vi "arm control.vi"(1 "State":T1, 2 "Z Axis (Tuning)":dbl) -> (0 "setpoint":dbl format="%.2f")   [LabVIEW 2013]
uses:
  typedefs/fg_typedef.ctl
  typedefs/subStates.ctl
panel:
  in  "lower limit":dbl=-0.015 format="%#_13g"
  in  "upper limit":dbl=0.015 format="%#_13g"
  in  "Up Setpoint":dbl format="%#_13g"
  # "Things needing Tuning"
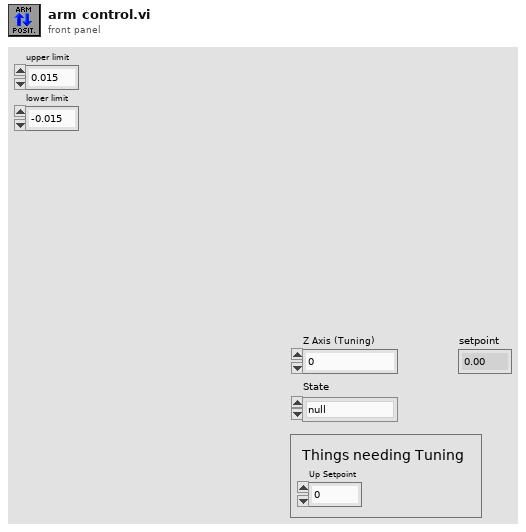
[diagram p1: front panel]
types:
  T1 = typedef "subStates.ctl" = enum16{"null", "wait", "driver control", "auto", "manual override", "hold position", "rotate", "pickup", "pass", "load", "goto shoot", "shoot high goal", "shoot low goal", "cancel arm", "cancel shooter", "end"}
  T2 = typedef "fg_typedef.ctl" = enum16{"Get", "Set"}
  T3 = typedef "WPI_DigitalInputDevRef.ctl" = cluster{"DevStatus":errorcluster, "DIO Channel":T4, "Digital Module":T5}
  T4 = typedef "FPGA_DIOChannel.ctl" = enum8{"DIO 1", "DIO 2", "DIO 3", "DIO 4", "DIO 5", "DIO 6", "DIO 7", "DIO 8", "DIO 9", "DIO 10", "DIO 11", "DIO 12", "DIO 13", "DIO 14", "Invalid"}
  T5 = typedef "FPGA_TypedefDigitalModule.ctl" = enum16{"Digital Module 1", "Digital Module 2"}
  T6 = typedef "WPI_EncoderDevRef.ctl" = cluster{"DevStatus":errorcluster, "EncoderIndex":T7, "CounterIndex":T8, "DistancePerCount":dbl, "Decoding Type":T9}
  T7 = typedef "FPGA_EncoderIdx.ctl" = enum8{"Enc 0", "Enc 1", "Enc 2", "Enc 3", "Invalid"}
  T8 = typedef "FPGA_CounterCtrSystemIndex.ctl" = enum8{"Ctr 0", "Ctr 1", "Ctr 2", "Ctr 3", "Ctr 4", "Ctr 5", "Ctr 6", "Ctr 7", "Invalid"}
  T9 = typedef "WPI_EncoderType.ctl" = enum16{"1x", "2x", "4x"}
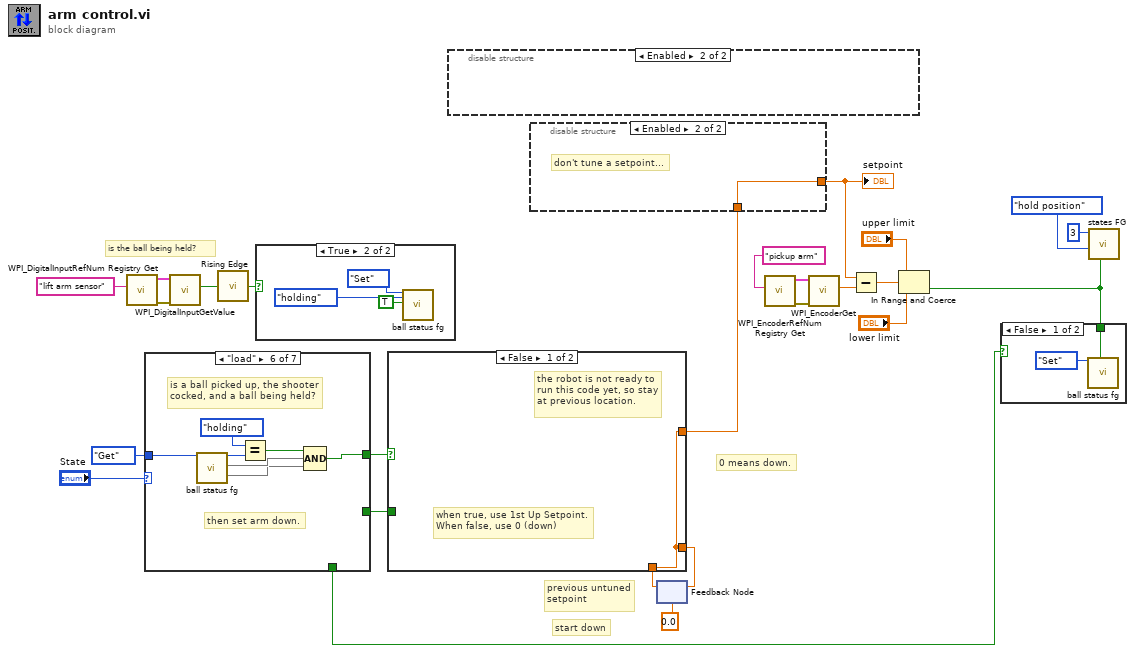
[diagram p0: block diagram]
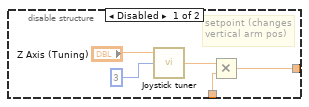
[diagram p3: hidden frame]
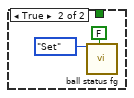
[diagram p4: hidden frame]
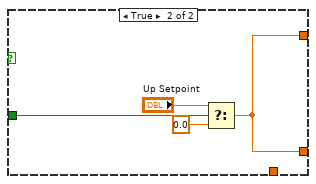
[diagram p6: hidden frame]
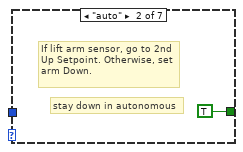
[diagram p8: hidden frame]
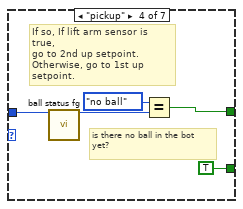
[diagram p10: hidden frame]
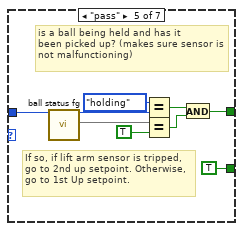
[diagram p11: hidden frame]
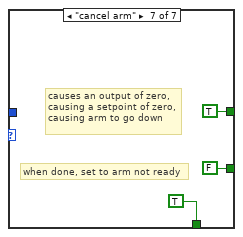
[diagram p12: hidden frame]
diagram:
  # "0 means down."
  # "is the ball being held?"
  # "start down"
  # "previous untuned\nsetpoint"
  n1 = call <vilib>:"WPI_DigitalInputRefNum Registry Get.vi"("refnum name"="lift arm sensor") -> ("error out"=w2:errorcluster, "DigitalInputDevRef"=w3:T3)  [unwired: 9 in]
  n2 = case shown="\"load\"" "State" {
    tunnel: fg_typedef."Get" ("Menu") -> [_ _ _ w31 w40 w47 _]
    tunnel: [_ TRUE _ w30 w35 w46 TRUE] -> w16
    tunnel: [_ _ _ TRUE ("y") TRUE ("y") _ FALSE ("y")] -> w15
    tunnel: [_ _ _ _ _ _ TRUE] -> w1
    frame "driver control", Default {
      # "code does not run"
    }
    frame "auto" {
      # "If lift arm sensor, go to 2nd\nUp Setpoint. Otherwise, set\narm Down."
      # "stay down in autonomous"
    }
    frame "manual override" {
      # "code does not run"
    }
    frame "pickup" {
      # "If so, If lift arm sensor is true,\ngo to 2nd up setpoint.\nOtherwise, go to 1st up\nsetpoint."
      # "is there no ball in the bot\nyet?"
      n3 = call "ball status fg.vi"("Menu"=w31) -> ("System State"=w28:enum16{"no ball", "holding", "loaded"})  [unwired: 18 in]
      n4 = Equal?(x=enum16{"no ball", "holding", "loaded"}."no ball" ("y"), y=w28) -> (x = y?=w30:bool)
    }
    frame "pass" {
      # "If so, if lift arm sensor is tripped,\ngo to 2nd up setpoint. Otherwise,\ngo to 1st Up setpoint."
      # "is a ball being held and has it\nbeen picked up? (makes sure sensor is\nnot malfunctioning)"
      n5 = call "ball status fg.vi"("Menu"=w40) -> ("System State"=w33:enum16{"no ball", "holding", "loaded"}, 16:w39)  [unwired: 17 in]
      n6 = Equal?(x=enum16{"no ball", "holding", "loaded"}."holding" ("y"), y=w33) -> (x = y?=w36:bool)
      n7 = Equal?(x=w39, y=TRUE) -> (x = y?=w37:bool)
      n8 = And(x=w36, y=w37) -> (x .and. y?=w35:bool)
    }
    frame "load" {
      # "then set arm down."
      # "is a ball picked up, the shooter\ncocked, and a ball being held?"
      n9 = call "ball status fg.vi"("Menu"=w47) -> ("System State"=w45:enum16{"no ball", "holding", "loaded"}, 16:w42, 18:w41)  [unwired: 16 in]
      n10 = Equal?(x=enum16{"no ball", "holding", "loaded"}."holding", y=w45) -> (x = y?=w43:bool)
      n11 = Compound Arithmetic op=AND(w43, w42, w41) -> (w46:bool)
    }
    frame "cancel arm" {
      # "when done, set to arm not ready"
      # "causes an output of zero,\ncausing a setpoint of zero,\ncausing arm to go down"
    }
  }
  n12 = call <vilib>:"WPI_DigitalInputGetValue.vi"("error in (no error)"=w2, "DigitalInputDevRef"=w3) -> ("Value"=w5:bool)  [unwired: 7 in, 2 out]
  n13 = call "Rising Edge.vi"("Input"=w5) -> ("Rising Edge"=w6:bool)
  n14 = case shown="True" w6 {
    frame False {
    }
    frame True {
      n15 = call "ball status fg.vi"("Menu"=fg_typedef."Set", "System State"=enum16{"no ball", "holding", "loaded"}."holding" ("Ball State Write"), 2:TRUE ("Picked Up")) -> ()  [unwired: 16 in, 1 out]
    }
  }
  n16 = disable-structure shown="Enabled" {
    frame Disabled {
      # "tuning value = coerce(.25, 1.5, ((Z -initZ)  * -1/2 + 1))"
      # "On first call, perform no tuning. Otherwise..."
    }
    frame Enabled {
    }
  }
  n17 = feedback #1(0.0 ("x")) -> (w8:dbl)
  n18 = case shown="False" w16 {
    tunnel: w15 -> [_ w56]
    tunnel: [w54 w55] -> w10
    tunnel: [w54 w55] -> w9
    tunnel: w8 -> [w54 _]
    frame False {
      # "when true, use 1st Up Setpoint.\nWhen false, use 0 (down)"
      # "the robot is not ready to\nrun this code yet, so stay\nat previous location."
    }
    frame True {
      n19 = Select(t="Up Setpoint", s=w56, f=0.0 ("x")) -> (s? t:f=w55:dbl)
    }
  }
  n20 = disable-structure shown="Enabled" {
    disable-tunnel: [w63 w64] -> w14
    disable-tunnel: w10 -> [w62 w64]
    frame Disabled {
      # "setpoint (changes\nvertical arm pos)"
      n21 = call "Joystick tuner.vi"("Joystick Z"="Z Axis (Tuning)", 2:3 ("Loop ID")) -> ("Output"=w61:dbl)  [unwired: 7 in]
      n22 = Multiply(x=w61, y=w62) -> (x*y=w63:dbl)
    }
    frame Enabled {
      # "don't tune a setpoint..."
    }
  }
  "setpoint" <- w14
  n23 = feedback-in #1(w9) -> ()
  n24 = call <vilib>:"WPI_EncoderRefNum Registry Get.vi"("refnum name"="pickup arm") -> ("error out"=w19:errorcluster, "EncoderDevRef"=w20:T6)  [unwired: 9 in]
  n25 = call <vilib>:"WPI_EncoderGet.vi"("error in (no error)"=w19, "EncoderDevRef"=w20) -> ("Distance"=w25:dbl)  [unwired: 4 in, 5 out]
  n26 = Subtract(x=w14, y=w25) -> (x-y=w22:dbl)
  n27 = In Range and Coerce(upper limit="upper limit", x=w22, lower limit="lower limit") -> (In Range?=w12:bool)  [unwired: 1 out]
  n28 = case shown="False" w1 {
    tunnel: w12 -> [w65 _]
    frame False {
      n29 = call "ball status fg.vi"("Menu"=fg_typedef."Set", 8:w65) -> ()  [unwired: 17 in, 1 out]
    }
    frame True {
      n30 = call "ball status fg.vi"("Menu"=fg_typedef."Set", 8:FALSE ("Arm Ready")) -> ()  [unwired: 17 in, 1 out]
    }
  }
  n31 = call "states FG.vi"("exit in"=w12, "subState in"=subStates."hold position", "Loop ID"=3) -> ()  [unwired: 5 in, 4 out]
